vi "Z900_navX_SERIAL_PacketChecksum.vi"(2 "error in (no error)":errorcluster, 3 "Packet":string) -> (0 "error out":errorcluster, 1 "Terminated Packet":string)   [LabVIEW 2019, in "navX Library v2.lvlib"]
uses:
  navX Library v2.lvlib
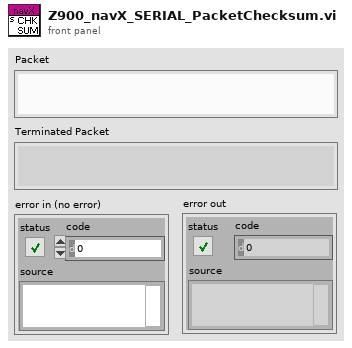
[diagram p1: front panel]
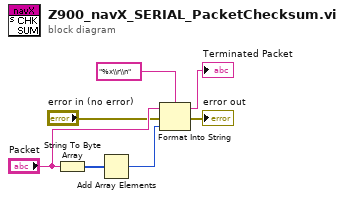
[diagram p0: block diagram]
diagram:
  n1 = String To Byte Array(string="Packet") -> (unsigned byte array=w5:u8[])
  n2 = Add Array Elements(numeric array=w5) -> (sum=w4:u8)
  n3 = Format Into String(format string="%x\\r\\n", initial string="Packet", error in="error in (no error)", w4) -> (resulting string=→"Terminated Packet":string, error out=→"error out":errorcluster)
